vi "_RT_CtrlLoop_D999_Conv_Switch_Value.vi"(1 "valid":bool, 3 "Response Str":string) -> (0 "switch array":bool[](array[boolean]))   [LabVIEW 2018]
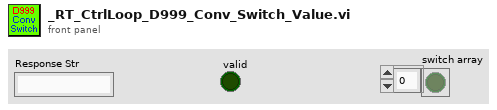
[diagram p1: front panel]
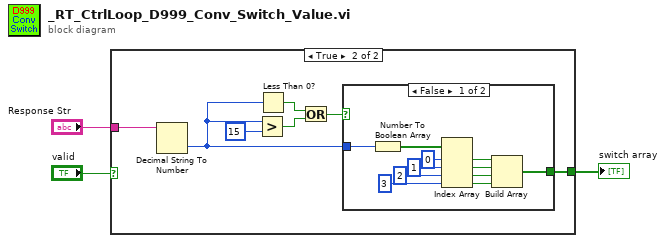
[diagram p0: block diagram]
diagram:
  n1 = case shown="True" "valid" {
    tunnel: [_ w10] -> w3
    tunnel: "Response Str" -> [_ w9]
    frame False {
    }
    frame True {
      n2 = Decimal String To Number(string=w9) -> (number=w8:i32)  [unwired: 2 in, 1 out]
      n3 = Greater?(x=w8, y=15) -> (0:w6:bool)
      n4 = Less Than 0?(x=w8) -> (x < 0?=w5:bool)
      n5 = Or(x=w5, y=w6) -> (x .or. y?=w4:bool)
      n6 = case shown="False" w4 {
        tunnel: [w12 _] -> w10
        tunnel: w8 -> [w11 _]
        frame False {
          n7 = Number To Boolean Array(number=w11) -> (Boolean array=w21:bool[])
          n8 = Index Array(array=w21, index #1=0 ("index"), index #2=1 ("index"), index #3=2 ("index"), index #4=3 ("index")) -> (element #1=w16:bool, element #2=w15:bool, element #3=w14:bool, element #4=w13:bool)
          n9 = Build Array(w16, w15, w14, w13) -> (w12:bool[])
        }
        frame True {
        }
      }
    }
  }
  "switch array" <- w3
